vi "read_file_as_line.vi"(0 "baud rate":u32=115200 caption="波特率", 1 "路径":path=path "C:/Users/Twsa/Documents/Graduction-Project/3Dprinter_labview/gcode_exe/file1.txt", 2 "端口":refnum<visa-resource-name>="COM4") -> ()   [LabVIEW 2018]
uses:
  <vilib>/Instr/_visa.llb/VISA Configure Serial Port (Instr).vi
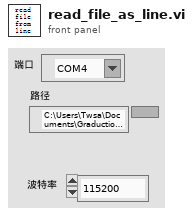
[diagram p1: front panel]
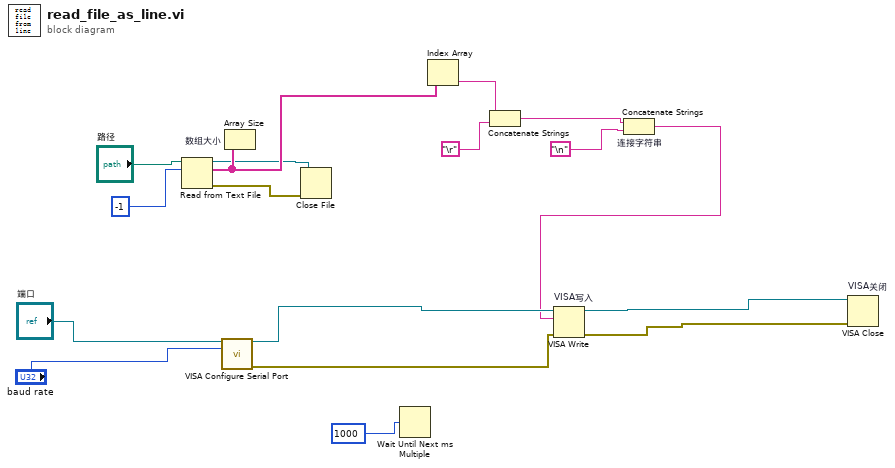
[diagram p0: block diagram]
diagram:
  n1 = Read from Text File(file (use dialog)="路径", count=-1) -> (refnum out=w13:refnum<file>, text=w15:string[], error out=w14:errorcluster)  [unwired: 2 in, 1 out]
  n2 = call-poly "VISA Configure Serial Port"("VISA resource name"="端口", "baud rate (9600)"="baud rate") -> ("VISA resource name out"=w9:refnum<visa-resource-name>, "error out"=w8:errorcluster)  [unwired: 12 in]
  n3 = Array Size "数组大小"(array=w15) -> ()  [unwired: 1 out]
  n4 = Close File(refnum=w13, error in=w14) -> ()  [unwired: 2 out]
  n5 = Wait Until Next ms Multiple(millisecond multiple=1000) -> ()  [unwired: 1 out]
  n6 = Index Array(array=w15) -> (element=w5:string)  [unwired: 1 in]
  n7 = Concatenate Strings(w5, "\r") -> (w2:string)
  n8 = Concatenate Strings "连接字符串"(w2, "\n") -> (w1:string)
  n9 = VISA Write "VISA写入"(VISA resource name=w9, write buffer=w1, error in (no error)=w8) -> (VISA resource name out=w11:refnum<visa-resource-name>, error out=w12:errorcluster)  [unwired: 1 out]
  n10 = VISA Close "VISA关闭"(VISA resource name=w11, error in (no error)=w12) -> ()  [unwired: 1 out]
